vi "csv_file_create.vi"(8 "error in (no error)":errorcluster, 11 "name or relative path":string="All NI Singapore Employees 2.csv") -> (0 "error out":errorcluster, 3 "Final Name List":string[](array[string]))   [LabVIEW 2018]
uses:
  <vilib>/Utility/file.llb/Read Delimited Spreadsheet (string).vi
  <vilib>/Utility/file.llb/Write Delimited Spreadsheet (string).vi
panel:
  out "Names portion":string[](array[string])
  out "all rows":string[][](array[string])
  out "Removed Header":string[][](array[string])
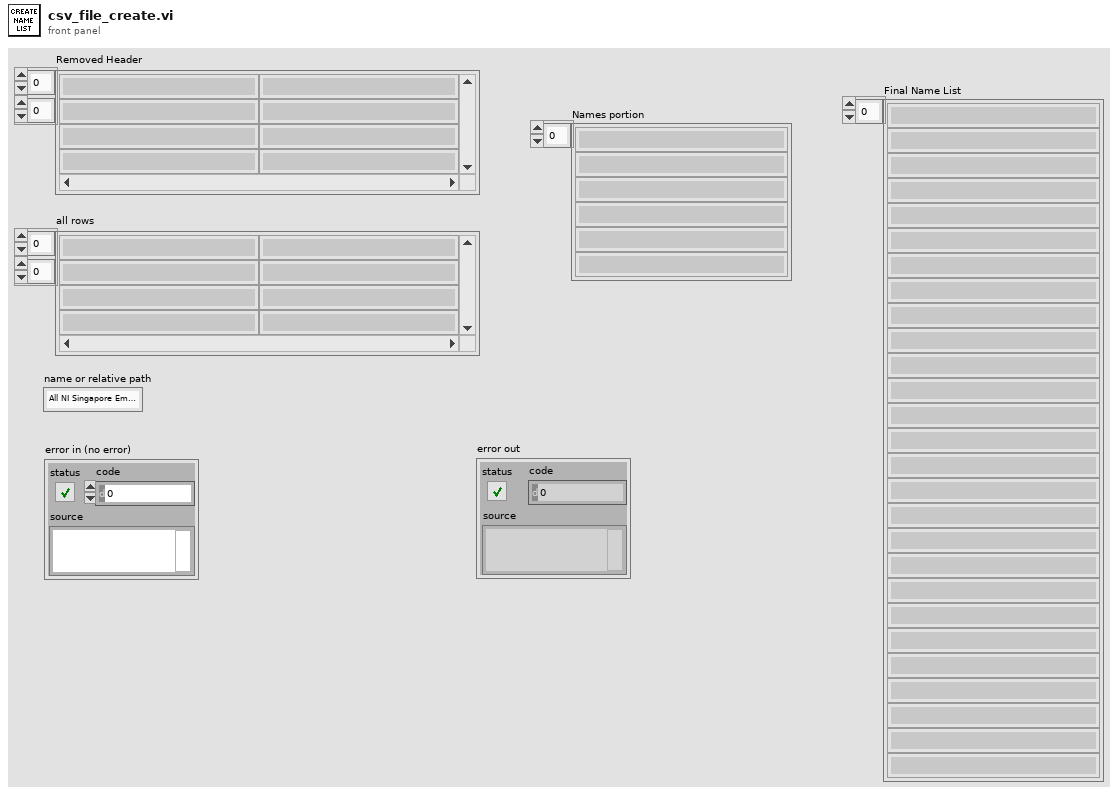
[diagram p1: front panel]
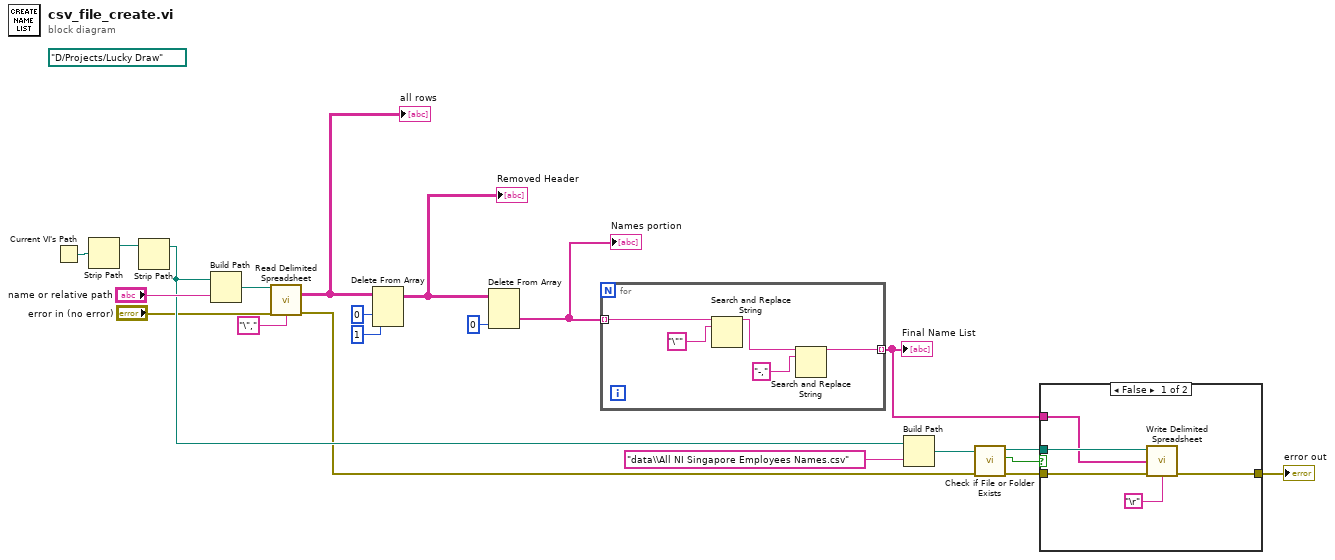
[diagram p0: block diagram]
diagram:
  (unwired) path "D:/Projects/Lucky Draw" ("base path")
  n1 = Current VI's Path() -> (path=w11:path)
  n2 = Strip Path(path=w11) -> (stripped path=w12:path)  [unwired: 1 out]
  n3 = Strip Path(path=w12) -> (stripped path=w10:path)  [unwired: 1 out]
  n4 = Build Path(base path=w10, name or relative path="name or relative path") -> (appended path=w20:path)
  n5 = call-poly <vilib>:"Read Delimited Spreadsheet.vi"("file path (dialog if empty)"=w20, "error in (no error)"="error in (no error)", "delimiter (\\t)"="\"," ("delimiter (\\t)")) -> ("all rows"=w16:string[][], "error out"=w7:errorcluster)  [unwired: 7 in, 4 out]
  "all rows" <- w16
  n6 = Delete From Array(array=w16, length=1, index (row)=0) -> (array with subset deleted=w15:string[][])  [unwired: 1 in, 1 out]
  "Removed Header" <- w15
  n7 = Delete From Array(array=w15, index (col)=0 ("disabled index (col)")) -> (deleted portion=w13:string[])  [unwired: 2 in, 1 out]
  "Names portion" <- w13
  n8 = for {
    tunnel: w13 -> [w26] mode=indexing
    tunnel: [w22] -> w3 mode=indexing
    n9 = Search and Replace String(input string=w26, search string="\"" ("input string")) -> (result string=w23:string)  [unwired: 6 in, 3 out]
    n10 = Search and Replace String(input string=w23, search string="-," ("input string")) -> (result string=w22:string)  [unwired: 6 in, 3 out]
  }
  "Final Name List" <- w3
  n11 = Build Path(base path=w10, name or relative path="data\\All NI Singapore Employees Names.csv") -> (appended path=w8:path)
  n12 = call <vilib>:"Check if File or Folder Exists.vi"("error in (no error)"=w7, "path"=w8) -> ("error out"=w6:errorcluster, "file or folder exists?"=w4:bool, "dup path"=w5:path)  [unwired: 7 in]
  n13 = case shown="False" w4 {
    tunnel: w6 -> [w31 w32]
    tunnel: w5 -> [w30 _]
    tunnel: w3 -> [w29 _]
    tunnel: [w27 w32] -> w1
    frame False {
      n14 = call-poly <vilib>:"Write Delimited Spreadsheet.vi"("file path (dialog if empty)"=w30, "1D data"=w29, "error in (no error)"=w31, "delimiter (\\t)"="\r") -> ("error out"=w27:errorcluster)  [unwired: 10 in, 1 out]
    }
    frame True {
    }
  }
  "error out" <- w1
